vi "Smite.vi"(8 "Error In":errorcluster, 11 "Selection List[]":refnum<vi>[](array[refnum])) -> (0 "Error Out":errorcluster, 3 "Change Made?":bool)   [LabVIEW 2017, in "Toolkit VIs.lvlib"]
doc: "Changes a grave site (Diagram Disable structure) to the Spirit frame (refactored code) and enables it. In other words, it smites zombie code."
uses:
  Toolkit VIs.lvlib
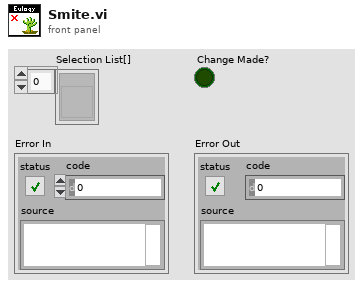
[diagram p1: front panel]
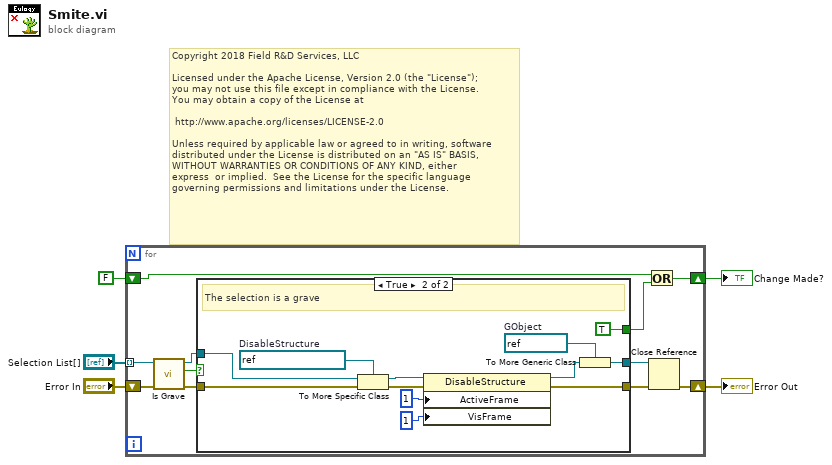
[diagram p0: block diagram]
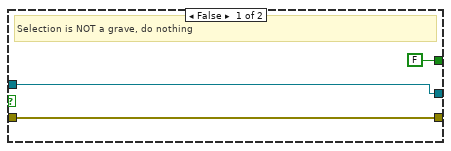
[diagram p2: hidden frame]
diagram:
  # "Copyright 2018 Field R&D Services, LLC\n\nLicensed under the Apache License, Version 2.0 (the \"License\");\nyou may not use this file except in compliance with the License.\nYou may obtain a copy of the License at\n\n\thttp://www.apache.org/licenses/LICENSE-2.0\n\nUnless required by applicable law or agreed to in writing, software\ndistributed under the License is distributed on an \"AS IS\" BASIS,\nWITHOUT WARRANTIES OR CONDITIONS OF ANY KIND, either \nexpress  or implied.  See the License for the specific language \ngoverning permissions and limitations under the License."
  n1 = for {
    shift-right: [w11] -> w5
    shift-left: "Error In" -> [w10]
    tunnel: "Selection List[]" -> [w7] mode=indexing
    shift-right: [w14] -> w3
    shift-left: FALSE -> [w16]
    n2 = call "Is Grave.vi"("Error In"=w10, "GObject In"=w7) -> ("Error Out"=w9:errorcluster, "Grave?"=w8:bool, "GObject Out"=w6:refnum<vi>)  [unwired: 7 in]
    n3 = case shown="True" w8 {
      tunnel: [FALSE ("y") TRUE ("y")] -> w15
      tunnel: [w17 w29] -> w13
      tunnel: [w18 w27] -> w12
      tunnel: w9 -> [w17 w25]
      tunnel: w6 -> [w18 w20]
      frame False {
        # "Selection is NOT a grave, do nothing"
      }
      frame True {
        w26 = refnum<vi> refnum  # GObject
        w31 = refnum<vi> refnum  # DisableStructure
        # "The selection is a grave"
        n4 = To More Specific Class(target class=w31, reference=w20, error in=w25) -> (specific class reference=w24:refnum<vi>, error out=w23:errorcluster)
        n5 = property class="DisableStructure"(reference=w24, error in=w23, "ActiveFrame"=i16 1 ("Active Frame"), "VisFrame"=u32 1 ("Visible Frame")) -> (reference out=w30:refnum<vi>, error out=w29:errorcluster)
        n6 = To More Generic Class(target class=w26, reference=w30) -> (generic class reference=w27:refnum<vi>)
      }
    }
    n7 = Or(x=w16, y=w15) -> (x .or. y?=w14:bool)
    n8 = Close Reference(reference=w12, error in (no error)=w13) -> (error out=w11:errorcluster)
  }
  "Error Out" <- w5
  "Change Made?" <- w3
